vi "GetThrottleReading.vi"(8 "error in":errorcluster, 10 "Channel Number (1-8)":T1=1 items=["Channel 1"=1, "Channel 2"=2, "Channel 3"=3, "Channel 4"=4, "Channel 5"=5, "Channel 6"=6, "Channel 7"=7, "Channel 8"=8], 11 "VISA resource name":refnum<visa-resource-name>) -> (0 "error out":errorcluster, 1 "Throttle reading":i8 format="%0.1f", 2 "Throttle reading string":string, 3 "VISA resource name out":refnum<visa-resource-name>)   [LabVIEW 2023, in "Thermotron 8800.lvlib"]
doc: "THTL\nCAUTION: Do not use the THTL command as an operation command. Using the THTL as an operation command overwrites 8800 internal control functions.\nCommand name: Send throttle reading\nCommand type: Variable\nDescription: The query command asks the 8800 for the current channel “n” throttle reading. The 8800 sends the throttle value as a percentage.\nSyntax: THTLn\nWhere n is any process variable channel (1 through 8).\nData type: Integer (-100 to +100)\nQuery example: THTL1?\n8800 response: -56 (The current throttle reading for process variable channel 1 is -56%.)"
uses:
  Thermotron 8800.lvlib
  Private/AnalogInputChannelNumber.ctl
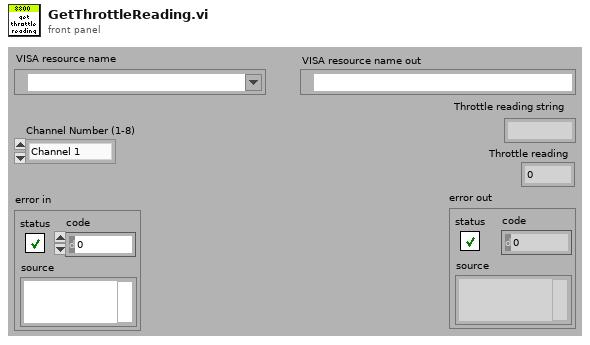
[diagram p1: front panel]
types:
  T1 = typedef "Thermotron 8800.lvlib/AnalogInputChannelNumber.ctl" = u16
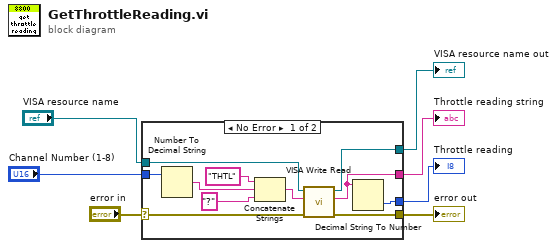
[diagram p0: block diagram]
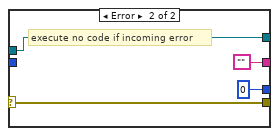
[diagram p2: hidden frame]
diagram:
  n1 = case shown="No Error" "error in" {
    selector: "error in" -> [w16 w21]
    tunnel: [w13 w21] -> w6
    tunnel: [w14 w22] -> w5
    tunnel: "VISA resource name" -> [w15 w22]
    tunnel: [w9 ""] -> w3
    tunnel: "Channel Number (1-8)" -> [w11 _]
    tunnel: [w8 0] -> w1
    frame No Error {
      n2 = Number To Decimal String(number=w11) -> (decimal integer string=w10:string)  [unwired: 1 in]
      n3 = Concatenate Strings("THTL" ("8800 Command"), w10, "?" ("8800 Command")) -> (w18:string)
      n4 = call "VISA Write Read.vi"("error in (no error)"=w16, "8800 Command"=w18, "VISA Refnum in"=w15) -> ("error out"=w13:errorcluster, "read buffer"=w9:string, "VISA Refnum out"=w14:refnum<visa-resource-name>)  [unwired: 6 in]
      n5 = Decimal String To Number(string=w9) -> (number=w8:i32)  [unwired: 2 in, 1 out]
    }
    frame Error {
      # "execute no code if incoming error"
    }
  }
  "VISA resource name out" <- w5
  "error out" <- w6
  "Throttle reading string" <- w3
  "Throttle reading" <- w1
